vi "FlatToRichrouteguide_request.vi"(5 "OutputClusterType":T1, 11 "InputCluster":T3) -> (3 "OutputCluster":T1)   [LabVIEW 2019, in "Generated_server.lvlib"]
uses:
  Generated_server.lvlib
  routeguide_request_Flat.ctl
  routeguide_Color.ctl
  routeguide_request.ctl
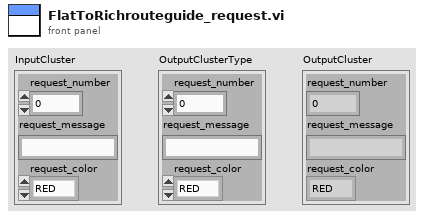
[diagram p1: front panel]
types:
  T1 = typedef "Generated_server.lvlib/routeguide_request.ctl" = cluster{"request_number":i32, "request_message":string, "request_color":T2}
  T2 = typedef "Generated_server.lvlib/routeguide_Color.ctl" = enum32{"RED", "GREEN", "BLUE"}
  T3 = typedef "Generated_server.lvlib/routeguide_request_Flat.ctl" = cluster{"request_number":i32, "request_message":string, "request_color":T2}
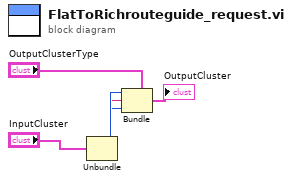
[diagram p0: block diagram]
diagram:
  n1 = Unbundle "Unbundle"("InputCluster") -> ("request_number"=w3:i32, "request_message"=w2:string, "request_color"=w1:T2)
  n2 = Bundle "Bundle"(cluster="OutputClusterType", "request_number"=w3, "request_message"=w2, "request_color"=w1) -> (→"OutputCluster":T1)
